vi "SaveToolTip.vi"(2 "ToolTip":cluster{"ToolTipOpen":bool, "LastToolTip":i32}, 5 "error in (no error)":errorcluster) -> (19 "error out":errorcluster)   [LabVIEW 2014, in "UmlEditor.lvclass"]
uses:
  <resource>/Framework/Providers/Open_GDS/UML/UmlEditor_class/UmlEditor.lvclass
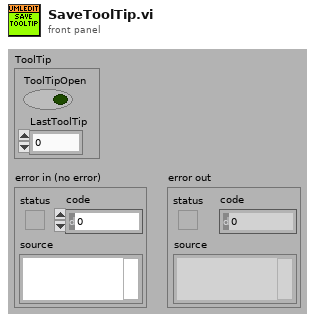
[diagram p1: front panel]
types:
  T1 = typedef "UmlEditor.lvclass/ObjectAttributes.ctl" = cluster{"ListeningQueueIn":refnum<queue>, "Event":refnum<user-event>, "UseProjectFolderAsBasePath":bool, "TypeSyncOption":bool, "Attr":string[], "ToolTip":cluster{"ToolTipOpen":bool, "LastToolTip":i32}, "ClassesToIgnore":string[], "UndoSize":i32, "OpenLastSavedFileWhenStarting":bool, "SyncOption":T2, "SyncTime(s)":i32, "Params":cluster{"IniParams":T3, "Value":string}[], "GraphButtons":refnum<vi>}
  T2 = typedef "UMLEditor_SyncOptions.ctl" = cluster{"IgnoreInstrLib":bool, "IgnoreUserLib":bool, "IgnoreViLib":bool}
  T3 = typedef "UmlEditor.lvclass/IniParamsType.ctl" = enum16{"I have problem with UML stability on my computer"}
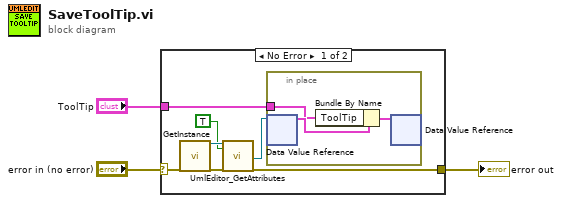
[diagram p0: block diagram]
diagram:
  n1 = case shown="No Error" "error in (no error)" {
    selector: "error in (no error)" -> [w8 w14]
    tunnel: [w7 w14] -> w2
    tunnel: "ToolTip" -> [w4 _]
    frame No Error {
      n2 = call <resource>:"GetInstance.vi"("error in (no error)"=w8) -> ("reference out"=w10:refnum<class "UmlEditor.lvclass">, "error out"=w9:errorcluster)  [unwired: 17 out]
      n3 = call <resource>:"UmlEditor_GetAttributes.vi"("reference in"=w10, "OnlyGetDvrReference(False)"=TRUE, "error in (no error)"=w9) -> ("DataRef"=w5:refnum<data-value>, "error out"=w7:errorcluster)  [unwired: 13 in, 2 out]
      n4 = in-place {
        in-place-border: w4 -> [w12]
        n5 = in-place-dvr #1(w5) -> (w13:T1)  [unwired: 1 out]
        n6 = Bundle By Name(cluster=w13, "ToolTip"=w12) -> (w11:T1)
        n7 = in-place-dvr #1(w11) -> ()  [unwired: 2 out]
      }
    }
    frame Error {
    }
  }
  "error out" <- w2
